vi "Configure Program Mode.vi"(0 "VISA resource name":refnum<visa-resource-name>, 3 "Single Step Mode (F:Disable)":bool, 5 "Loop Cycle (1)":i32=1 min=0 max=9999 step=1, 11 "error in (no error)":errorcluster, 14 "Enable Over Current Fold Back (F:Disable)":bool) -> (4 "VISA resource name out":refnum<visa-resource-name>, 15 "error out":errorcluster)   [LabVIEW 2016, in "APT 300XAC Series.lvlib"]
doc: "Sets the instrument in program mode and configures the parameters in it.\n\nIn the program mode the instrument can be programmed for a sequence of operations/Settings with the help of a list of 50 sequential memories with 9 steps each. Each step can be configured with user configurable testing parameters such as test time, high and low limits, etc."
uses:
  APT 300XAC Series.lvlib
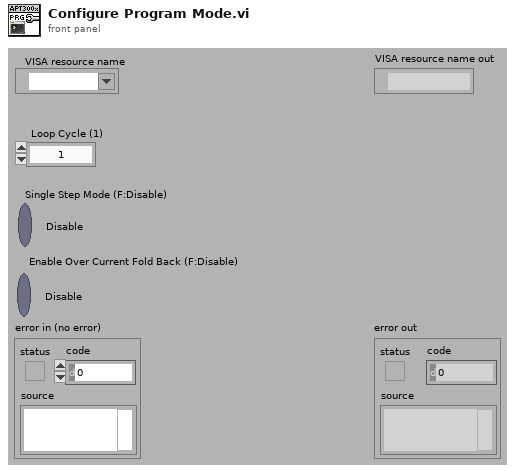
[diagram p1: front panel]
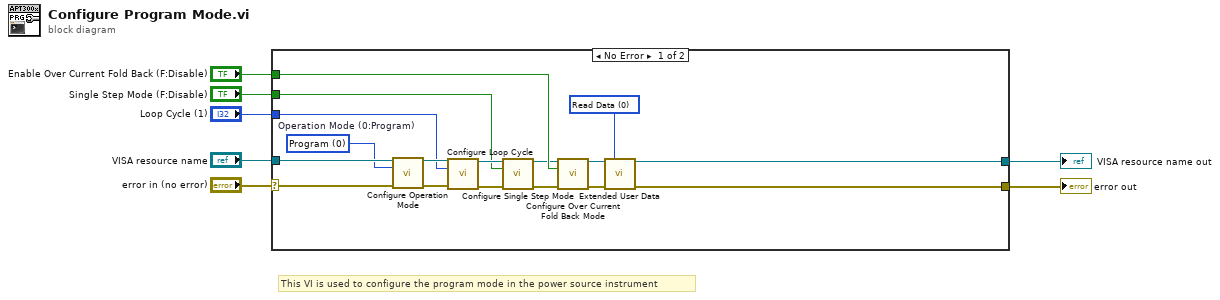
[diagram p0: block diagram]
diagram:
  # "This VI is used to configure the program mode in the power source instrument"
  n1 = case shown="No Error" "error in (no error)" {
    selector: "error in (no error)" -> [w19 w26]
    tunnel: [w10 w26] -> w7
    tunnel: [w11 w25] -> w6
    tunnel: "VISA resource name" -> [w20 w25]
    tunnel: "Loop Cycle (1)" -> [w18 _]
    tunnel: "Single Step Mode (F:Disable)" -> [w17 _]
    tunnel: "Enable Over Current Fold Back (F:Disable)" -> [w16 _]
    frame No Error {
      w8 = u16 0 items=["Read Data", "Write Data", "Clear Data", "Clear ALL Data"] ("Action")
      w13 = u16 0 items=["Program", "Manual", "DC+", "DC-"]  # Operation Mode (0:Program)
      n2 = call "Configure Operation Mode.vi"("VISA resource name"=w20, "Operation Mode (0:Program)"=w13, "error in (no error)"=w19) -> ("VISA resource name out"=w21:refnum<visa-resource-name>, "error out"=w22:errorcluster)  [unwired: 11 in]
      n3 = call "Configure Loop Cycle.vi"("VISA resource name"=w21, "Loop Cycle (1)"=w18, "error in (no error)"=w22) -> ("VISA resource name out"=w23:refnum<visa-resource-name>, "error out"=w24:errorcluster)  [unwired: 11 in]
      n4 = call "Configure Single Step Mode.vi"("VISA resource name"=w23, "Single Step Mode (F:Disable)"=w17, "error in (no error)"=w24) -> ("VISA resource name out"=w15:refnum<visa-resource-name>, "error out"=w14:errorcluster)  [unwired: 11 in]
      n5 = call "Configure Over Current Fold Back Mode.vi"("VISA resource name"=w15, "Enable Over Current Fold Back (F:Disable)"=w16, "error in (no error)"=w14) -> ("VISA resource name out"=w12:refnum<visa-resource-name>, "error out"=w9:errorcluster)  [unwired: 11 in]
      n6 = call "Extended User Data.vi"("VISA resource name"=w12, "Action"=w8, "Error In (no error)"=w9) -> ("VISA resource name out"=w11:refnum<visa-resource-name>, "Error Out"=w10:errorcluster)  [unwired: 10 in, 1 out]
    }
    frame Error {
    }
  }
  "error out" <- w7
  "VISA resource name out" <- w6
